vi "Paused Control Logic.vi"(8 "error in (no error)":errorcluster, 10 "parameters in":T1, 11 "Sequencer Module runtime in":refnum<class "Sequencer Module runtime.lvclass">) -> (0 "error out":errorcluster, 2 "parameters out":T1, 3 "Sequencer Module runtime out":refnum<class "Sequencer Module runtime.lvclass">)   [LabVIEW 2015, in "Sequencer Module runtime.lvclass"]
doc: "This Vi Controls the Actions Available in the Pause State\nStart which resumes the sequence"
uses:
  Sequencer Module runtime.lvclass
  <vilib>/NI/Tag Bus/table/data table.ctl
  Sequencer State Enum.ctl
  Sequencer Module runtime.lvclass/Sequencer Module runtime.ctl
  <vilib>/NI/Tag Bus/table/data table.lvlib
panel:
  # "Manual Input"
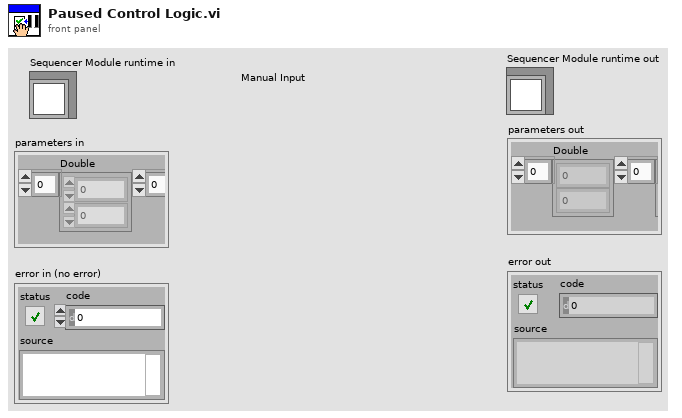
[diagram p1: front panel]
types:
  T1 = typedef "tag bus.lvlib/data table.lvlib/data table.ctl" = cluster{"Double":dbl[], "Single":sgl[], "I64":i64[], "I32":i32[], "I16":i16[], "I8":i8[], "U64":u64[], "U32":u32[], "U16":u16[], "U8":u8[], "Boolean":bool[], "String":string[], "Array of Double":cluster{"DBL Array":dbl[]}[], "Array of Single":cluster{"SGL Array":sgl[]}[], "Array of I64":cluster{"I64 Array":i64[]}[], "Array of I32":cluster{"I32 Array":i32[]}[], "Array of I16":cluster{"I16 Array":i16[]}[], "Array of I8":cluster{"I8 Array":i8[]}[], "Array of U64":cluster{"U64 Array":u64[]}[], "Array of U32":cluster{"U32 Array":u32[]}[], "Array of U16":cluster{"U16 Array":u16[]}[], "Array of U8":cluster{"U8 Array":u8[]}[], "Array of Boolean":cluster{"Boolean Array":bool[]}[], "Array of String":cluster{"String Array":string[]}[]}
  T2 = typedef "Sequencer Module runtime.lvclass/Sequencer Control.ctl" = cluster{"Start":bool, "Change Sequence":bool, "New Sequence":i32, "Pause":bool, "Abort":bool, "Terminate":bool}
  T3 = typedef "Sequencer Module runtime.lvclass/Sequencer State Enum.ctl" = enum16{"Idle", "Paused", "Start Sequence", "Run Sequence", "CleanUp Sequence", "Generate Report"}
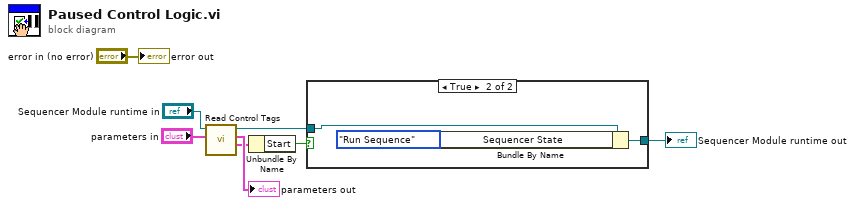
[diagram p0: block diagram]
diagram:
  n1 = call "Read Control Tags.vi"("Paramaters  allocation in"="parameters in", "Sequencer Module runtime in"="Sequencer Module runtime in") -> ("Sequence Control"=w2:T2, "Parameters allocation out"=→"parameters out":T1, "Sequencer Module runtime out"=w5:refnum<class "Sequencer Module runtime.lvclass">)  [unwired: 7 in]
  n2 = Unbundle By Name(w2) -> ("Start"=w1:bool)
  n3 = case shown="True" w1 {
    tunnel: w5 -> [w9 w12]
    tunnel: [w9 w11] -> w8
    frame False {
    }
    frame True {
      n4 = Bundle By Name(cluster=w12, "Sequencer State"=Sequencer_State_Enum."Run Sequence" ("Sequencer State.Sequencer State")) -> (w11:refnum<class "Sequencer Module runtime.lvclass">)
    }
  }
  "Sequencer Module runtime out" <- w8
  "error out" <- "error in (no error)"
